vi "Find RF In-Out Re-Patch Places.vi"(10 "TestSequence":T1[](array[typedef])) -> (2 "TestSequence out":T1[](array[typedef]))   [LabVIEW 2017]
doc: "Detect where to prompt the operator to connect the APAR RF in or RF out connector to the PNA. Do this at sequence start time and put the property into the sequence structure that gets executed."
uses:
  TestStep-StepType.ctl
  TestStepTypes.ctl
  RF Direction.ctl
  PolarizationSelect.ctl
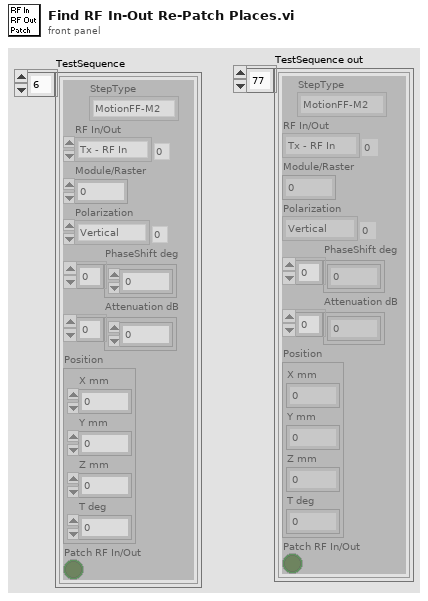
[diagram p1: front panel]
types:
  T1 = typedef "TestStep-StepType.ctl" = cluster{"StepType":T2, "RF In/Out":T3, "Module/Raster":i32, "Polarization":T4, "PhaseShift deg":dbl[], "Attenuation dB":dbl[], "Position":cluster{"X mm":dbl, "Y mm":dbl, "Z mm":dbl, "T deg":dbl}, "Patch RF In/Out":bool}
  T2 = typedef "TestStepTypes.ctl" = enum16{"MotionFF-M2", "Motion", "SweepTest", "RasterTest", "Finish", "64ModuleCfg"}
  T3 = typedef "RF Direction.ctl" = enum16{"Tx - RF In", "Rx - RF Out"}
  T4 = typedef "PolarizationSelect.ctl" = enum16{"Vertical", "Horizontal"}
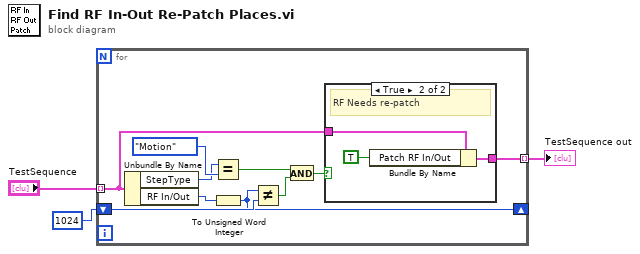
[diagram p0: block diagram]
diagram:
  n1 = for {
    shift-right: [w4] -> _
    shift-left: u16 1024 -> [w10]
    tunnel: "TestSequence" -> [w7] mode=indexing
    tunnel: [w5] -> w1 mode=indexing
    n2 = Unbundle By Name(w7) -> ("StepType"=w8:T2, "RF In/Out"=w9:T3)
    n3 = Equal?(x=w8, y=TestStepTypes."Motion" ("StepType")) -> (x = y?=w11:bool)
    n4 = To Unsigned Word Integer(number=w9) -> (unsigned 16bit integer=w4:u16)
    n5 = Not Equal?(x=w4, y=w10) -> (x != y?=w12:bool)
    n6 = And(x=w11, y=w12) -> (x .and. y?=w6:bool)
    n7 = case shown="True" w6 {
      tunnel: w7 -> [w14 w17]
      tunnel: [w14 w15] -> w5
      frame False {
      }
      frame True {
        # "RF Needs re-patch"
        n8 = Bundle By Name(cluster=w17, "Patch RF In/Out"=TRUE) -> (w15:T1)
      }
    }
  }
  "TestSequence out" <- w1
